vi "Post-Build Action.vi"(5 "Files Generated by Build":path[](array[path]), 6 "Top Level/Always Included VIs":path[](array[path]), 7 "Destination Path":path, 8 "error in (no error)":errorcluster, 9 "Target Name":string, 10 "Build Specification Name":string, 11 "Project Path":path) -> (0 "error out":errorcluster)   [LabVIEW 2020]
uses:
  <vilib>/MeasurementLink/LabVIEW Measurement Service Template/RPC Messages/ni_measurementlink_measurement_v1_MeasurementDetails.ctl
  <vilib>/Utility/config.llb/Write Key (String).vi
  <vilib>/Utility/config.llb/NI_LVConfig.lvlib
  <vilib>/MeasurementLink/LabVIEW Measurement Service Template/MeasurementTemplate_server-release.lvlib
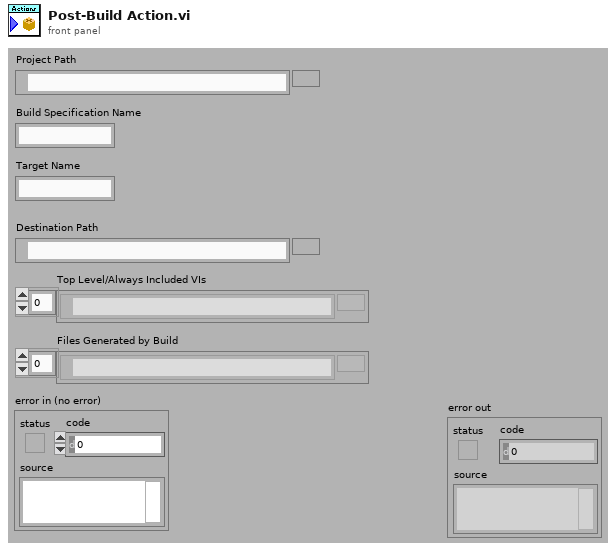
[diagram p1: front panel]
types:
  T1 = cluster{"Target Name":string, "Top Level/Always Included VIs":path[], "Project Path":path, "Destination Path":path, "Build Specification Name":string, "Files Generated by Build":path[]}
  T2 = typedef "MeasurementTemplate_server-release.lvlib/ni_measurementlink_measurement_v1_MeasurementDetails.ctl" = cluster{"display_name":string, "version":string}
  T3 = cluster{"displayName":string, "serviceClass":string, "providedInterfaces":string[], "path":string, "descriptionUrl":string}
  T4 = cluster{"services":cluster{"displayName":string, "serviceClass":string, "providedInterfaces":string[], "path":string, "descriptionUrl":string}[]}
  T5 = cluster{"displayName":string, "serviceClass":string, "providedInterfaces":string[], "path":string, "descriptionUrl":string}[]
  T6 = typedef "NI_LVConfig.lvlib/Config Data RefNum.ctl" = refnum<k1>
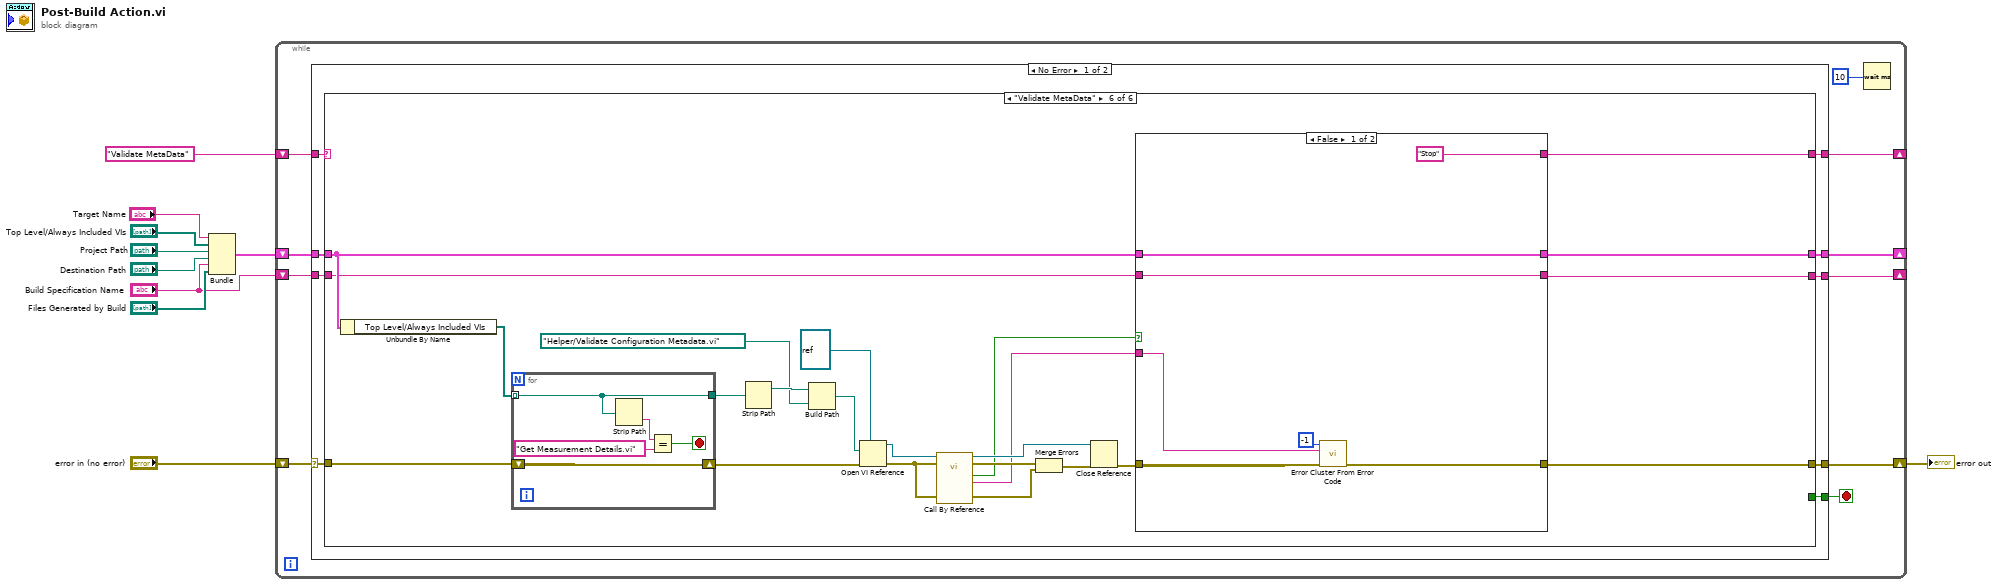
[diagram p0: block diagram]
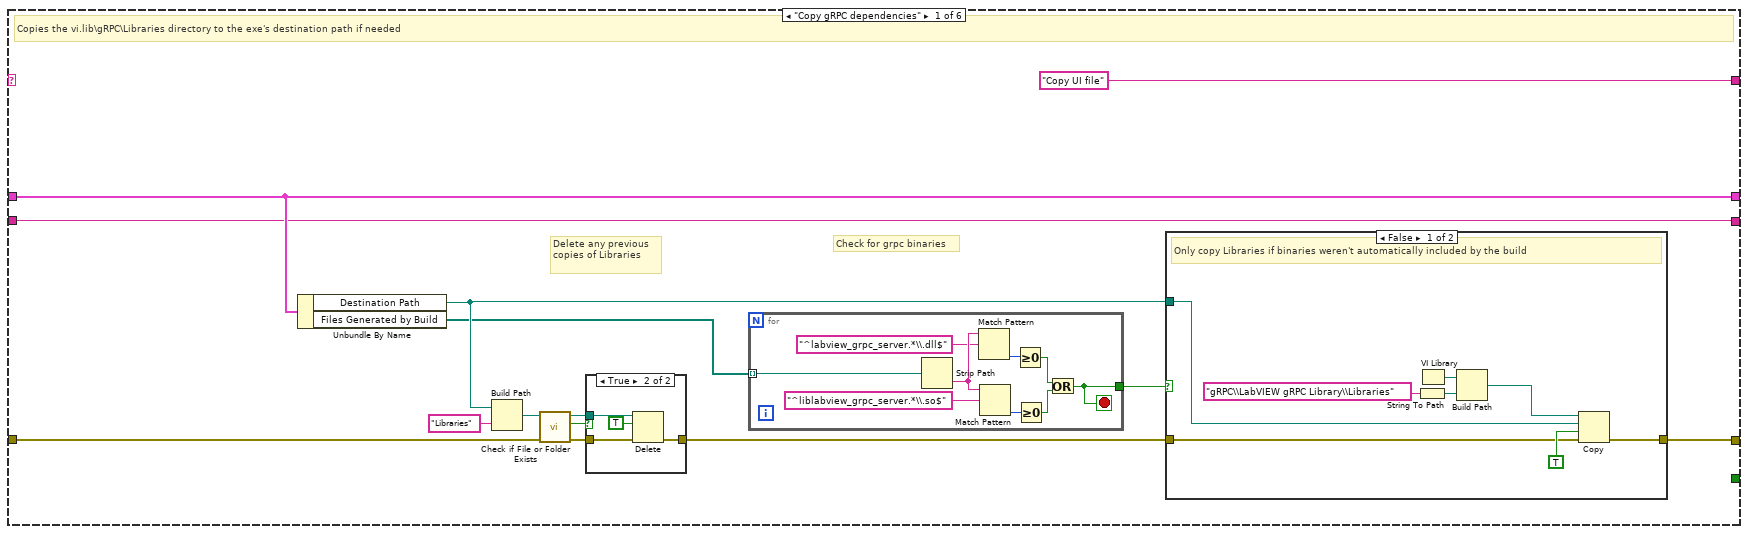
[diagram p2: hidden frame]
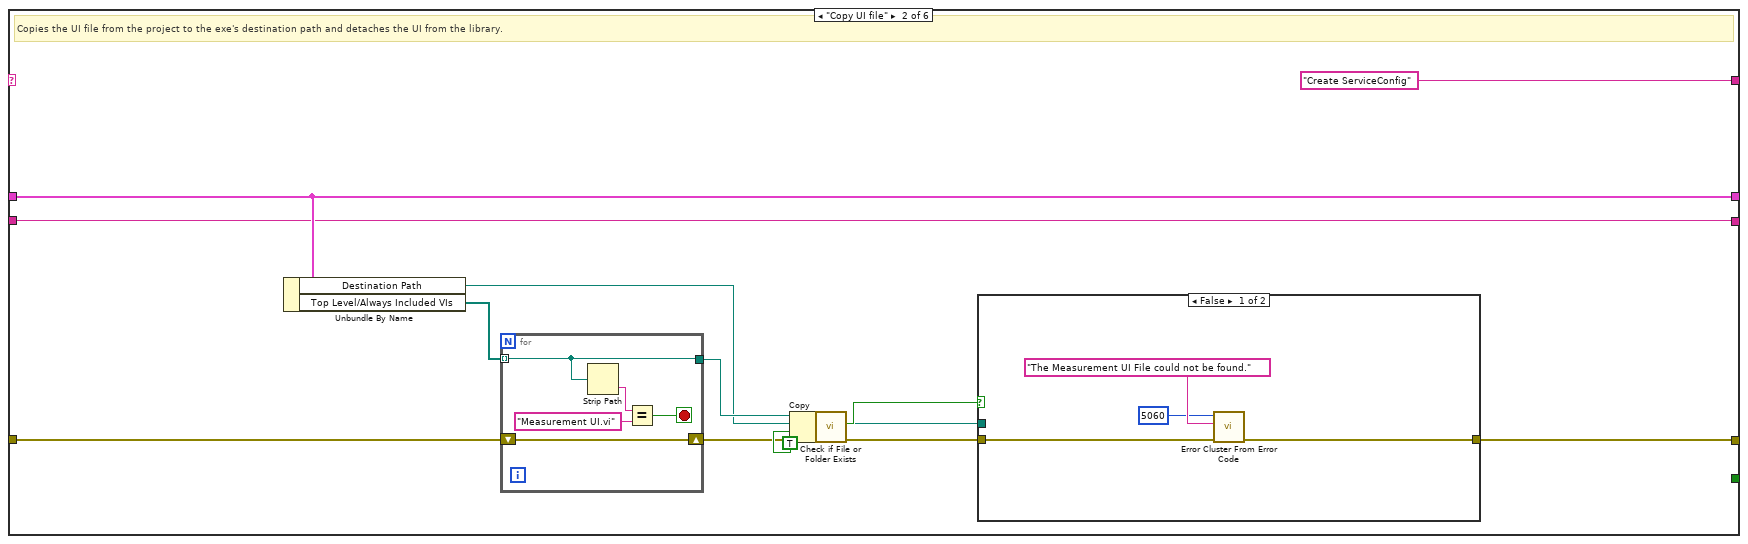
[diagram p5: hidden frame]
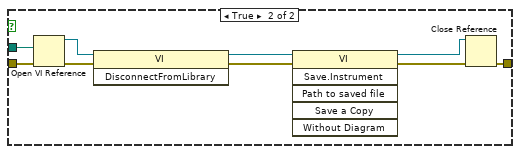
[diagram p6: hidden frame]
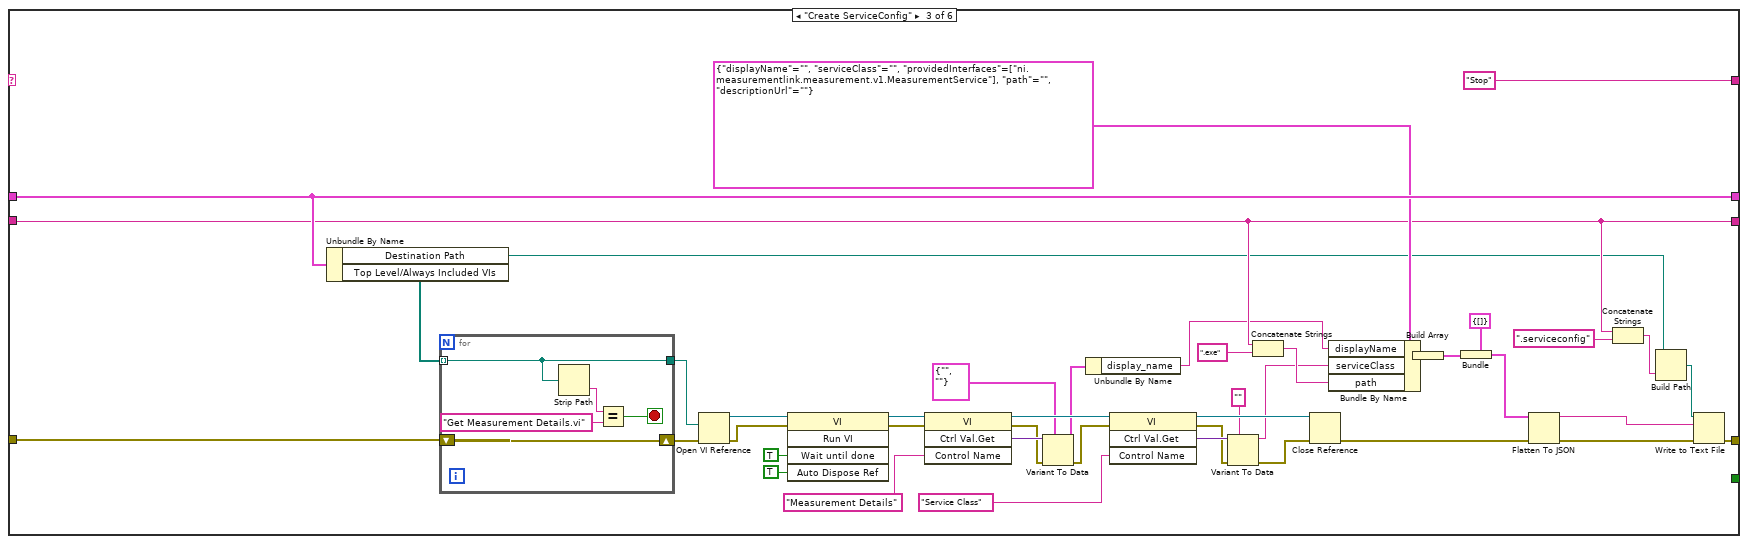
[diagram p7: hidden frame]
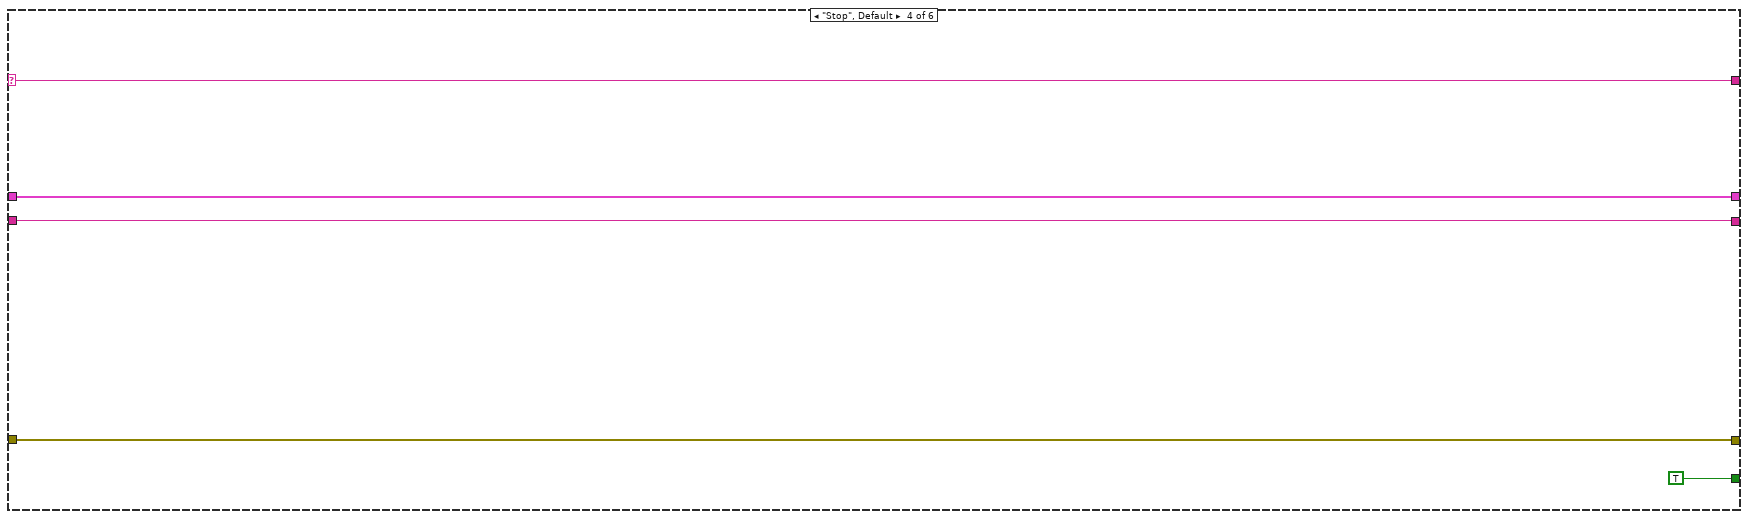
[diagram p8: hidden frame]
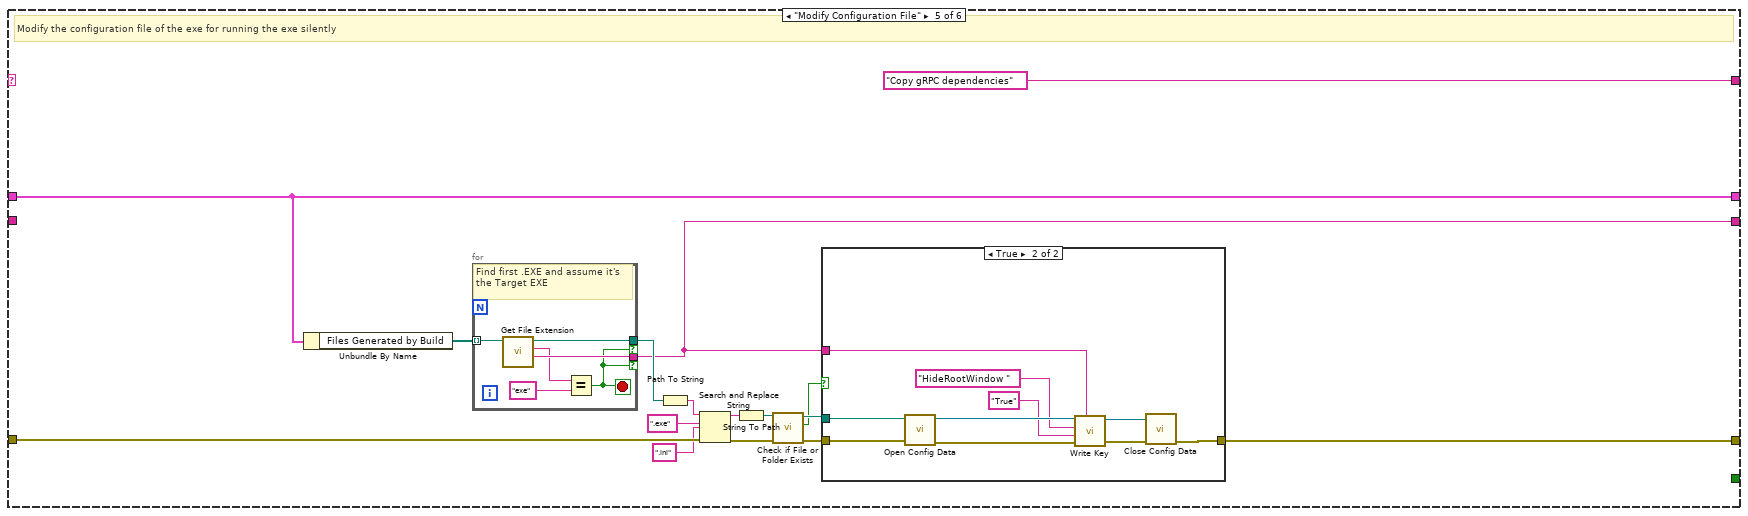
[diagram p9: hidden frame]
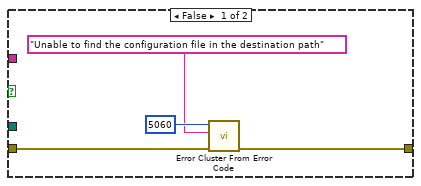
[diagram p10: hidden frame]
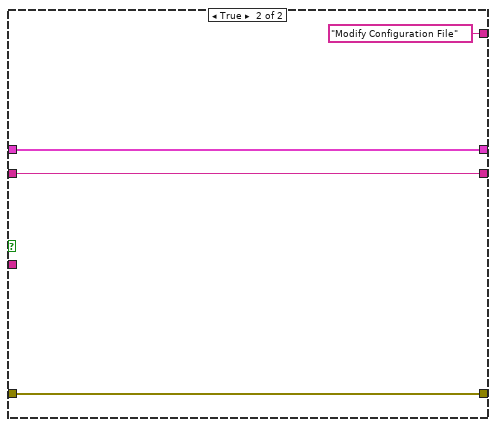
[diagram p11: hidden frame]
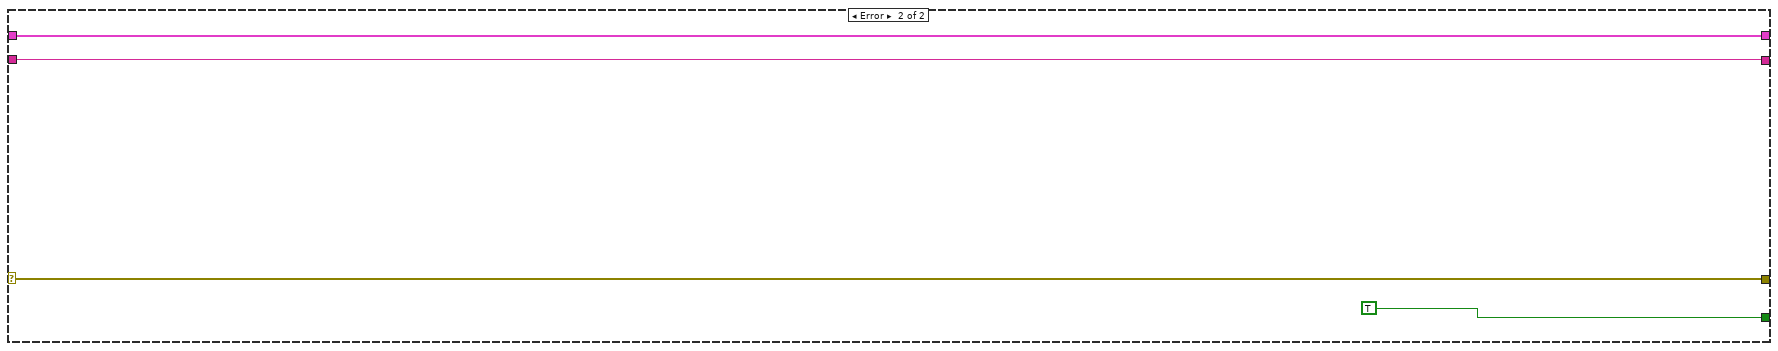
[diagram p12: hidden frame]
diagram:
  n1 = Bundle("Target Name"="Target Name", "Top Level/Always Included VIs"="Top Level/Always Included VIs", "Project Path"="Project Path", "Destination Path"="Destination Path", "Build Specification Name"="Build Specification Name", "Files Generated by Build"="Files Generated by Build") -> (w4:T1)  [unwired: 1 in]
  n2 = while {
    shift-right: [w17] -> _
    shift-left: w4 -> [w18]
    shift-right: [w16] -> w2
    shift-left: "error in (no error)" -> [w13]
    shift-right: [w15] -> _
    shift-left: "Validate MetaData" -> [w19]
    shift-right: [w12] -> _
    shift-left: "Build Specification Name" -> [w11]
    stop <- w14 stop-if-true
    n3 = case shown="No Error" w13 {
      selector: w13 -> [w23 w230]
      tunnel: w19 -> [w29 _]
      tunnel: w18 -> [w28 w231]
      tunnel: [w27 w231] -> w17
      tunnel: [w26 w230] -> w16
      tunnel: [w25 _] -> w15
      tunnel: [w24 TRUE] -> w14
      tunnel: [w22 w228] -> w12
      tunnel: w11 -> [w21 w228]
      frame No Error {
        n4 = case shown="\"Validate MetaData\"" w29 {
          selector: w29 -> [_ _ _ w150 _ _]
          tunnel: w28 -> [w41 w81 w141 w152 w164 w193]
          tunnel: [w41 w81 w141 w152 w164 w192] -> w27
          tunnel: w23 -> [w33 w73 w140 w149 w162 w198]
          tunnel: [w43 w78 w105 w149 w168 w211] -> w26
          tunnel: ["Copy UI file" "Create ServiceConfig" "Stop" w150 "Copy gRPC dependencies" w189] -> w25
          tunnel: [_ _ _ TRUE _ _] -> w24
          tunnel: [w40 w67 w111 w148 w154 w190] -> w22
          tunnel: w21 -> [w40 w67 w111 w148 _ w191]
          frame "Copy gRPC dependencies" {
            # "Delete any previous copies of Libraries"
            # "Check for grpc binaries"
            # "Copies the vi.lib\\gRPC\\Libraries directory to the exe's destination path if needed"
            n5 = Unbundle By Name(w41) -> ("Destination Path"=w32:path, "Files Generated by Build"=w30:path[])
            n6 = Build Path(base path=w32, name or relative path="Libraries") -> (appended path=w38:path)
            n7 = call <vilib>:"Check if File or Folder Exists.vi"("error in (no error)"=w33, "path"=w38) -> ("error out"=w37:errorcluster, "file or folder exists?"=w35:bool, "dup path"=w36:path)  [unwired: 7 in]
            n8 = case shown="True" w35 {
              tunnel: w37 -> [w53 w57]
              tunnel: [w53 w56] -> w31
              tunnel: w36 -> [_ w54]
              frame False {
              }
              frame True {
                n9 = Delete(path (use dialog)=w54, entire hierarchy (F)=TRUE ("confirm (F)"), error in=w57) -> (error out=w56:errorcluster)  [unwired: 2 in, 2 out]
              }
            }
            n10 = for {
              tunnel: [w44] -> w39
              tunnel: w30 -> [w49] mode=indexing
              stop <- w44 stop-if-true
              n11 = Strip Path(path=w49) -> (name=w52:string)  [unwired: 1 out]
              n12 = Match Pattern(string=w52, regular expression="^labview_grpc_server.*\\.dll$" ("pattern")) -> (offset past match=w48:i32)  [unwired: 1 in, 3 out]
              n13 = Match Pattern(string=w52, regular expression="^liblabview_grpc_server.*\\.so$" ("pattern")) -> (offset past match=w47:i32)  [unwired: 1 in, 3 out]
              n14 = Greater Or Equal To 0?(x=w48) -> (x >= 0?=w46:bool)
              n15 = Greater Or Equal To 0?(x=w47) -> (x >= 0?=w45:bool)
              n16 = Or(x=w46, y=w45) -> (x .or. y?=w44:bool)
            }
            n17 = case shown="False" w39 {
              tunnel: [w61 w66] -> w43
              tunnel: w32 -> [w59 _]
              tunnel: w31 -> [w58 w66]
              frame False {
                # "Only copy Libraries if binaries weren't automatically included by the build"
                n18 = String To Path(string="gRPC\\LabVIEW gRPC Library\\Libraries") -> (path=w63:path)
                n19 = VI Library() -> (path=w65:path)
                n20 = Build Path(base path=w65, name or relative path=w63) -> (appended path=w62:path)
                n21 = Copy(8:w58, 9:TRUE ("overwrite (F)"), 10:w59, 11:w62) -> (0:w61:errorcluster)  [unwired: 1 in, 2 out]
              }
              frame True {
              }
            }
          }
          frame "Copy UI file" {
            # "Copies the UI file from the project to the exe's destination path and detaches the UI from the library."
            n22 = Unbundle By Name(w81) -> ("Destination Path"=w74:path, "Top Level/Always Included VIs"=w76:path[])
            n23 = for {
              tunnel: w76 -> [w97] mode=indexing
              tunnel: [w97] -> w75
              shift-right: [w95] -> w72
              shift-left: w73 -> [w95]
              stop <- w98 stop-if-true
              n24 = Strip Path(path=w97) -> (name=w99:string)  [unwired: 1 out]
              n25 = Equal?(x=w99, y="Measurement UI.vi") -> (x = y?=w98:bool)
            }
            n26 = Copy(8:w72, 9:TRUE ("overwrite (F)"), 10:w74, 11:w75) -> (0:w80:errorcluster, 3:w70:path)  [unwired: 1 in, 1 out]
            n27 = call <vilib>:"Check if File or Folder Exists.vi"("error in (no error)"=w80, "path"=w70) -> ("error out"=w71:errorcluster, "file or folder exists?"=w69:bool, "dup path"=w68:path)  [unwired: 7 in]
            n28 = case shown="False" w69 {
              tunnel: w71 -> [w85 w94]
              tunnel: [w84 w90] -> w78
              tunnel: w68 -> [_ w89]
              frame False {
                n29 = call <vilib>:"Error Cluster From Error Code.vi"("error in (no error)"=w85, "error message (\"\")"="The Measurement UI File could not be found." ("error message (\"\")"), "error code (0)"=5060) -> ("error out"=w84:errorcluster)  [unwired: 6 in]
              }
              frame True {
                n30 = Open VI Reference(vi path=w89, error in (no error)=w94) -> (vi reference=w91:refnum<vi>, error out=w93:errorcluster)  [unwired: 4 in]
                n31 = invoke class="VI" method="DisconnectFromLibrary"(reference=w91, error in=w93) -> (reference out=w87:refnum<vi>, error out=w92:errorcluster)  [unwired: 1 in, 1 out]
                n32 = invoke class="VI" method="Save.Instrument"(reference=w87, error in=w92) -> (reference out=w86:refnum<vi>, error out=w88:errorcluster)  [unwired: 4 in, 4 out]
                n33 = Close Reference(reference=w86, error in (no error)=w88) -> (error out=w90:errorcluster)
              }
            }
          }
          frame "Create ServiceConfig" {
            n34 = Unbundle By Name(w141) -> ("Destination Path"=w109:path, "Top Level/Always Included VIs"=w142:path[])
            n35 = for {
              tunnel: w142 -> [w145] mode=indexing
              tunnel: [w145] -> w139
              shift-right: [w143] -> w138
              shift-left: w140 -> [w143]
              stop <- w146 stop-if-true
              n36 = Strip Path(path=w145) -> (name=w147:string)  [unwired: 1 out]
              n37 = Equal?(x=w147, y="Get Measurement Details.vi") -> (x = y?=w146:bool)
            }
            n38 = Open VI Reference(vi path=w139, error in (no error)=w138) -> (vi reference=w137:refnum<vi>, error out=w129:errorcluster)  [unwired: 4 in]
            n39 = invoke class="VI" method="Run VI"(reference=w137, error in=w129, "Wait until done"=TRUE ("Wait Until Done"), "Auto Dispose Ref"=TRUE ("Auto Dispose Reference")) -> (reference out=w134:refnum<vi>, error out=w130:errorcluster)  [unwired: 1 in, 3 out]
            n40 = invoke class="VI" method="Ctrl Val.Get"(reference=w134, error in=w130, "Control Name"="Measurement Details") -> (reference out=w131:refnum<vi>, error out=w125:errorcluster, "Get Control Value Variant"=w126:variant)  [unwired: 1 in, 1 out]
            n41 = Variant To Data(error in=w125, type=T2 {"display_name"="", "version"=""} ("ni_measurements_v1_MeasurementDetails"), Variant=w126) -> (data=w114:T2, error out=w124:errorcluster)
            n42 = Unbundle By Name(w114) -> ("display_name"=w101:string)
            n43 = invoke class="VI" method="Ctrl Val.Get"(reference=w131, error in=w124, "Control Name"="Service Class") -> (reference out=w128:refnum<vi>, error out=w122:errorcluster, "Get Control Value Variant"=w123:variant)  [unwired: 1 in, 1 out]
            n44 = Variant To Data(error in=w122, type="", Variant=w123) -> (data=w100:string, error out=w121:errorcluster)
            n45 = Concatenate Strings(w111, ".exe" ("string")) -> (w102:string)
            n46 = Close Reference(reference=w128, error in (no error)=w121) -> (error out=w107:errorcluster)
            n47 = Bundle By Name(cluster=T3 {"displayName"="", "serviceClass"="", "providedInterfaces"=["ni.measurementlink.measurement.v1.MeasurementService"], "path"="", "descriptionUrl"=""}, "displayName"=w101, "serviceClass"=w100, "path"=w102) -> (w116:T3)
            n48 = Build Array(w116) -> (w115:T5)
            n49 = Bundle(cluster=T4 {"services"=[]}, "services"=w115) -> (w113:T4)
            n50 = Flatten To JSON(anything=w113, error in (no error)=w107) -> (JSON string=w112:string, 11:w106:errorcluster)  [unwired: 1 in]
            n51 = Concatenate Strings(w111, ".serviceconfig" ("string")) -> (w108:string)
            n52 = Build Path(base path=w109, name or relative path=w108) -> (appended path=w104:path)
            n53 = Write to Text File(file (use dialog)=w104, text=w112, error in=w106) -> (error out=w105:errorcluster)  [unwired: 1 in, 2 out]
          }
          frame "Stop", Default {
          }
          frame "Modify Configuration File" {
            # "Modify the configuration file of the exe for running the exe silently"
            n54 = Unbundle By Name(w164) -> ("Files Generated by Build"=w163:path[])
            n55 = for {
              tunnel: w163 -> [w174] mode=indexing
              tunnel: [w173] -> w154 if=w169
              tunnel: [w172] -> w156 if=w169
              stop <- w169 stop-if-true
              # "Find first .EXE and assume it's the Target EXE"
              n56 = call <vilib>:"Get File Extension.vi"("file"=w174) -> ("filename without extension"=w173:string, "lowercase file extension"=w170:string, "dup file"=w172:path)  [unwired: 6 in, 2 out]
              n57 = Equal?(x=w170, y="exe") -> (x = y?=w169:bool)
            }
            n58 = Path To String(path=w156) -> (string=w155:string)
            n59 = Search and Replace String(input string=w155, search string=".exe", replace string=".ini", error in=w162) -> (result string=w159:string, error out=w161:errorcluster)  [unwired: 4 in, 2 out]
            n60 = String To Path(string=w159) -> (path=w158:path)
            n61 = call <vilib>:"Check if File or Folder Exists.vi"("error in (no error)"=w161, "path"=w158) -> ("error out"=w167:errorcluster, "file or folder exists?"=w165:bool, "dup path"=w166:path)  [unwired: 7 in]
            n62 = case shown="True" w165 {
              tunnel: [w177 w188] -> w168
              tunnel: w166 -> [_ w181]
              tunnel: w167 -> [w178 w180]
              tunnel: w154 -> [_ w179]
              frame False {
                n63 = call <vilib>:"Error Cluster From Error Code.vi"("error in (no error)"=w178, "error message (\"\")"="Unable to find the configuration file in the destination path" ("source"), "error code (0)"=5060) -> ("error out"=w177:errorcluster)  [unwired: 6 in]
              }
              frame True {
                n64 = call <vilib>:"Open Config Data.vi"("error in (no error)"=w180, "configuration file path"=w181) -> ("error out"=w187:errorcluster, "refnum"=w186:T6)  [unwired: 7 in, 1 out]
                n65 = call-poly <vilib>:"Write Key.vi"("section"=w179, "error in (no error)"=w187, "value"="True", "key"="HideRootWindow ", "refnum"=w186) -> ("error out"=w184:errorcluster, "refnum out"=w183:T6)  [unwired: 4 in, 1 out]
                n66 = call <vilib>:"Close Config Data.vi"("error in (no error)"=w184, "refnum"=w183) -> ("error out"=w188:errorcluster)  [unwired: 8 in, 1 out]
              }
            }
          }
          frame "Validate MetaData" {
            n67 = Unbundle By Name(w193) -> ("Top Level/Always Included VIs"=w210:path[])
            n68 = for {
              tunnel: w210 -> [w214] mode=indexing
              tunnel: [w214] -> w207
              shift-right: [w212] -> w206
              shift-left: w198 -> [w212]
              stop <- w215 stop-if-true
              n69 = Strip Path(path=w214) -> (name=w216:string)  [unwired: 1 out]
              n70 = Equal?(x=w216, y="Get Measurement Details.vi") -> (x = y?=w215:bool)
            }
            n71 = Strip Path(path=w207) -> (stripped path=w209:path)  [unwired: 1 out]
            n72 = Build Path(base path=w209, name or relative path=path "Helper/Validate Configuration Metadata.vi") -> (appended path=w205:path)
            n73 = Open VI Reference(type specifier VI Refnum (for type only)=refnum<vi> refnum, vi path=w205, error in (no error)=w206) -> (vi reference=w204:refnum<vi>, error out=w202:errorcluster)  [unwired: 3 in]
            n74 = call-by-ref "?"(reference=w204, error in=w202, 8:"error in (no error)"=w202) -> (reference out=w203:refnum<vi>, error out=w201:errorcluster, 0:"error out"=w199:errorcluster, "Invalid Parameters"=w196:string, "Is Metadata Valid"=w197:bool)  [unwired: 8 in]
            n75 = Merge Errors(w201, w199) -> (w200:errorcluster)
            n76 = Close Reference(reference=w203, error in (no error)=w200) -> (error out=w195:errorcluster)
            n77 = case shown="False" w197 {
              tunnel: w195 -> [w220 w227]
              tunnel: [w219 w227] -> w211
              tunnel: w196 -> [w217 _]
              tunnel: w193 -> [w223 w226]
              tunnel: [w223 w226] -> w192
              tunnel: w191 -> [w222 w225]
              tunnel: [w222 w225] -> w190
              tunnel: ["Stop" "Modify Configuration File"] -> w189
              frame False {
                n78 = call <vilib>:"Error Cluster From Error Code.vi"("error in (no error)"=w220, "error message (\"\")"=w217, "error code (0)"=-1) -> ("error out"=w219:errorcluster)  [unwired: 6 in]
              }
              frame True {
              }
            }
          }
        }
      }
      frame Error {
      }
    }
    n79 = Wait (ms)(milliseconds to wait=u32 10 ("millisecond timer value")) -> ()  [unwired: 1 out]
  }
  "error out" <- w2
